vi "Get Location of next IFD.vi"(4 "Litt/BigEnd":bool, 5 "Start of current IFD\n(ImFileDirectOffs)":i32, 8 "Image Data":u8[](array[numeric])) -> (0 "Location in byte stream of Long Word that points to this next IFD":i32, 3 "Location in byte stream of next IFD if there is a next IFD,\n0 otherwise":u32)   [LabVIEW 2013, in "Tiff reader.lvlib"]
doc: "Obtains the location of the pointer that points to the next IFD location. It also returns the destination of the pointer, the location of the next IFD.\n\n(Inlined to prevent extra array copies)"
uses:
  Tiff reader.lvlib
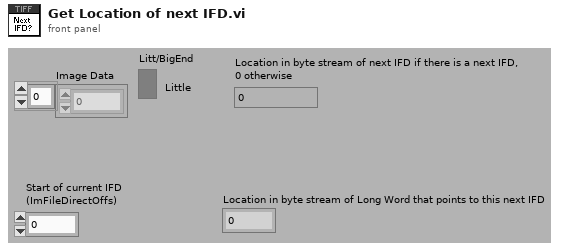
[diagram p1: front panel]
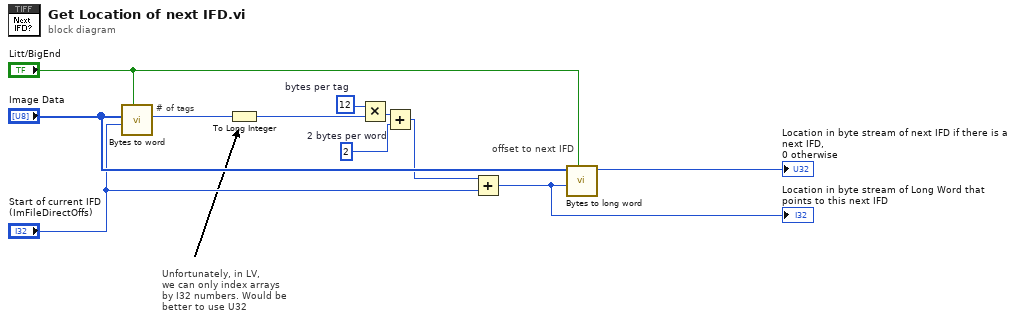
[diagram p0: block diagram]
diagram:
  w4 = 2  # 2 bytes per word
  w5 = 12  # bytes per tag
  # "Unfortunately, in LV,\nwe can only index arrays\nby I32 numbers. Would be\nbetter to use U32"
  # "offset to next IFD"
  # "# of tags"
  n1 = call "Bytes to word.vi"("Litt/BigEnd"="Litt/BigEnd", "Index"="Start of current IFD\n(ImFileDirectOffs)", "Image Data in"="Image Data") -> ("Word"=w3:u16)  [unwired: 1 in, 5 out]
  n2 = To Long Integer(number=w3) -> (32bit integer=w2:i32)
  n3 = Multiply(x=w5, y=w2) -> (x*y=w6:i32)
  n4 = Add(x=w6, y=w4) -> (x+y=w1:i32)
  n5 = Add(x=w1, y="Start of current IFD\n(ImFileDirectOffs)") -> (x+y=w11:i32)
  "Location in byte stream of Long Word that points to this next IFD" <- w11
  n6 = call "Bytes to long word.vi"("Litt/BigEnd"="Litt/BigEnd", "Index"=w11, "Image Data in"="Image Data") -> ("U32"=→"Location in byte stream of next IFD if there is a next IFD,\n0 otherwise":u32)  [unwired: 6 out]
